vi "RotateColorNTimes.vi"() -> ()   [LabVIEW 2019]
uses:
  Placeholder_Colors.ctl
panel:
  in  "Temp":T1
  in  "Start_Color":T1
  in  "Num Rotations":dbl
  # "TEMP VALUE FOR SENSOR CHANGE TO SENSOR VALUE"
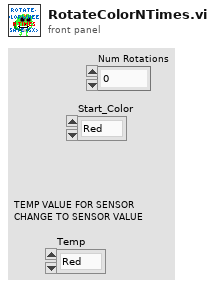
[diagram p1: front panel]
types:
  T1 = typedef "Placeholder_Colors.ctl" = enum16{"Red", "Yellow", "Blue", "Green", "Unknown"}
  T2 = typedef "WPI_MotorControlDeviceRef.ctl" = cluster{"DeviceStatus":errorcluster, "Type":T3, "PWM":cluster{"PWM Channel":T4, "DeadBand":T5}, "CAN":cluster{"Device Number":u8, "SetOutput VI Ref":variant, "GetOutput VI Ref":variant, "Enable VI Ref":variant, "Disable VI Ref":variant, "Data":variant}, "Invert":bool, "DIO PWM":cluster{"PWM \"Enable\" Channel":T4, "DIOChannel":T6, "PWM Rate":dbl}}
  T3 = typedef "WPI_MotorControlType.ctl" = enum16{"PWM", "CAN", "DIO PWM"}
  T4 = typedef "FPGA_DIOPWMChannel.ctl" = enum8{"PWM 0", "PWM 1", "PWM 2", "PWM 3", "PWM 4", "PWM 5", "PWM 6", "PWM 7", "PWM 8", "PWM 9", "PWM MXP 0", "PWM MXP 1", "PWM MXP 2", "PWM MXP 3", "PWM MXP 4", "PWM MXP 5", "PWM MXP 6", "PWM MXP 7", "PWM MXP 8", "PWM MXP 9", "Invalid"}
  T5 = typedef "WPI_PWMDeadband.ctl" = cluster{"Name":string, "maxPositivePwm":i32, "minPositivePwm":i32, "centerPwm":i32, "maxNegativePwm":i32, "minNegativePwm":i32, "angularRange":u16}
  T6 = typedef "FPGA_DIOChannel.ctl" = enum8{"DIO 0", "DIO 1", "DIO 2", "DIO 3", "DIO 4", "DIO 5", "DIO 6", "DIO 7", "DIO 8", "DIO 9", "DIO MXP 0", "DIO MXP 1", "DIO MXP 2", "DIO MXP 3", "DIO MXP 4", "DIO MXP 5", "DIO MXP 6", "DIO MXP 7", "DIO MXP 8", "DIO MXP 9", "DIO MXP 10", "DIO MXP 11", "DIO MXP 12", "DIO MXP 13", "DIO MXP 14", "DIO MXP 15", "SPI Port CS1", "SPI Port CS2", "SPI Port CS3", "SPI Port MISO", "SPI Port MOSI", "Invalid"}
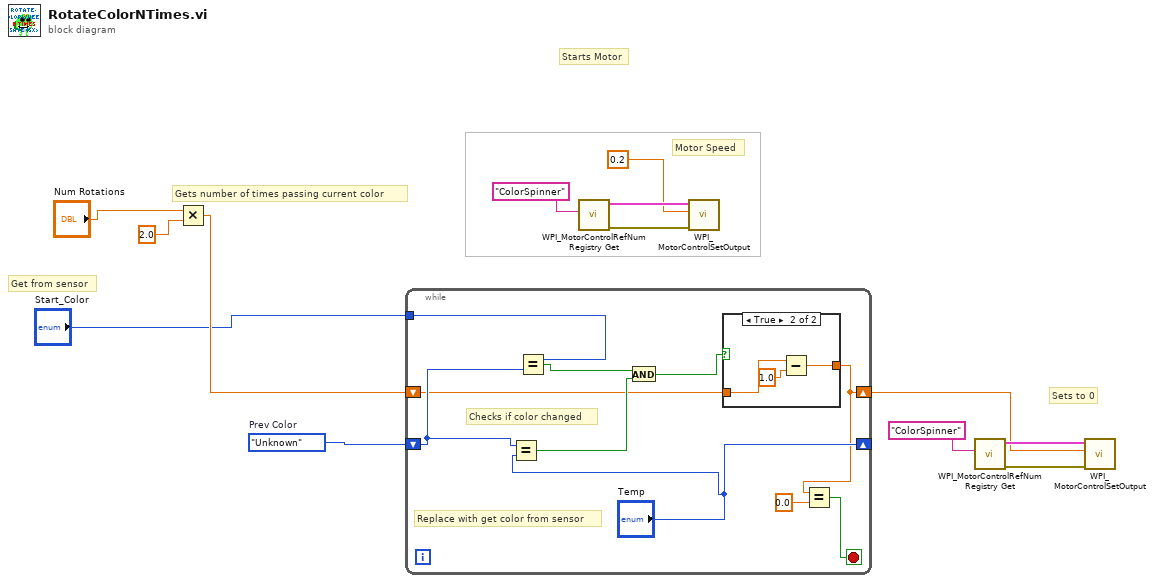
[diagram p0: block diagram]
diagram:
  w10 = Placeholder_Colors."Unknown"  # Prev Color
  # "Sets to 0"
  # "Get from sensor"
  # "Motor Speed"
  # "Starts Motor"
  # "Gets number of times passing current color"
  n1 = Multiply(x="Num Rotations", y=2.0) -> (x*y=w11:dbl)
  n2 = while {
    shift-right: [w16] -> w5
    shift-left: w11 -> [w18]
    shift-right: ["Temp"] -> _
    shift-left: w10 -> [w21]
    tunnel: "Start_Color" -> [w23]
    stop <- w14 stop-if-true
    # "Checks if color changed"
    # "Replace with get color from sensor"
    n3 = Equal?(x=w21, y="Temp") -> (x = y?=w20:bool)
    n4 = Equal?(x=w23, y=w21) -> (x = y?=w22:bool)
    n5 = And(x=w22, y=w20) -> (x .and. y?=w19:bool)
    n6 = case shown="True" w19 {
      tunnel: w18 -> [_ w26]
      tunnel: [_ w24] -> w16
      frame False {
      }
      frame True {
        n7 = Subtract(x=w26, y=1.0) -> (x-y=w24:dbl)
      }
    }
    n8 = Equal?(x=w16, y=0.0) -> (x = y?=w14:bool)
  }
  n9 = call <vilib>:"WPI_MotorControlRefNum Registry Get.vi"("refnum name"="ColorSpinner") -> ("error out"=w4:errorcluster, "MotorControlDevRef"=w3:T2)  [unwired: 9 in]
  n10 = call <vilib>:"WPI_MotorControlSetOutput.vi"("error in (no error)"=w4, "Output"=0.2, "MotorControlDevRef"=w3) -> ()  [unwired: 6 in, 3 out]
  n11 = call <vilib>:"WPI_MotorControlRefNum Registry Get.vi"("refnum name"="ColorSpinner") -> ("error out"=w8:errorcluster, "MotorControlDevRef"=w7:T2)  [unwired: 9 in]
  n12 = call <vilib>:"WPI_MotorControlSetOutput.vi"("error in (no error)"=w8, "Output"=w5, "MotorControlDevRef"=w7) -> ()  [unwired: 6 in, 3 out]
